vi "Timer.vi"(11 "Set Time [s]":dbl) -> (1 "Time elapsed!":bool, 3 "Elapsed time [s]":dbl)   [LabVIEW 2016]
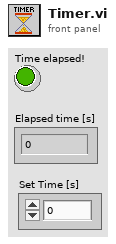
[diagram p1: front panel]
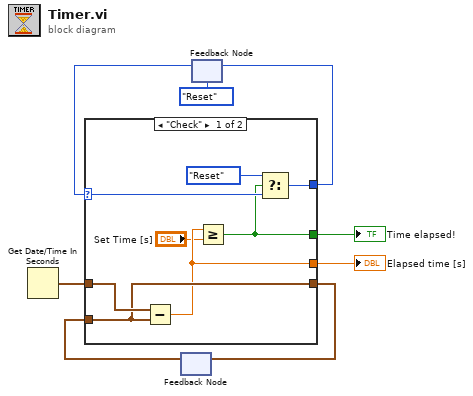
[diagram p0: block diagram]
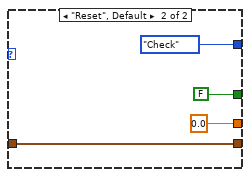
[diagram p2: hidden frame]
diagram:
  n1 = Get Date/Time In Seconds() -> (seconds since 1Jan1904=w6:timestamp)
  n2 = feedback #1() -> (w1:timestamp)  [unwired: 1 in]
  n3 = feedback #2(enum16{"Check", "Reset"}."Reset") -> (w4:enum16{"Check", "Reset"})
  n4 = case shown="\"Check\"" w4 {
    selector: w4 -> [w11 _]
    tunnel: [w15 w19] -> w2
    tunnel: [w14 0.0] -> w7
    tunnel: w6 -> [w16 w19]
    tunnel: w1 -> [w15 _]
    tunnel: [w10 enum16{"Check", "Reset"}."Check"] -> w3
    tunnel: [w9 FALSE] -> w8
    frame "Check" {
      n5 = Subtract(x=w16, y=w15) -> (x-y=w14:dbl)
      n6 = Greater Or Equal?(x=w14, y="Set Time [s]") -> (x >= y?=w9:bool)
      n7 = Select(t=enum16{"Check", "Reset"}."Reset", s=w9, f=w11) -> (s? t:f=w10:enum16{"Check", "Reset"})
    }
    frame "Reset", Default {
    }
  }
  "Time elapsed!" <- w8
  "Elapsed time [s]" <- w7
  n8 = feedback-in #1(w2) -> ()
  n9 = feedback-in #2(w3) -> ()
